vi "Set_Setting.vi"(5 "ChangeonFly":T4, 8 "SettingsCluster":T2={"Sample Rate (us)"=1, "Samples Per Data Point (int, power of 2)"=1000, "DistanceToBulk (um)"=-1.0, "HoldTimeScaler"=1, "SaveData"=TRUE, "DistanceToBulk (um) 2"=-1.0, "DistanceToBulk (um) 3"=-1.0}, 9 "VelScallerCluster":T3, 11 "FPGA VI Reference Out 2":T1) -> (0 "FPGAAccumulatorLength_inpowersof2":i16, 3 "FPGA VI Reference Out 4":T1)   [LabVIEW 2023]
uses:
  TypeDefs/ChangeOnFly.ctl
  TypeDefs/VelScallerCluster.ctl
  TypeDefs/Settings.ctl
  TypeDefs/FPGA VI reference.ctl
  User_Vi/Settings.vi
  <vilib>/Utility/error.llb/Error Cluster From Error Code.vi
  <vilib>/rvi/errors/niLvFpgaAdjustHostInterfaceError.vi
  <vilib>/rvi/interface/nirviReadWriteControl/nirviReadWriteControl.xnode
  FPGA Bitfiles/wecspmpcie7856mi_FPGATarget2_FPGATargetPCIe78_PFpA9M1zUPQ.lvbitx
  NiFpgaLv.dll
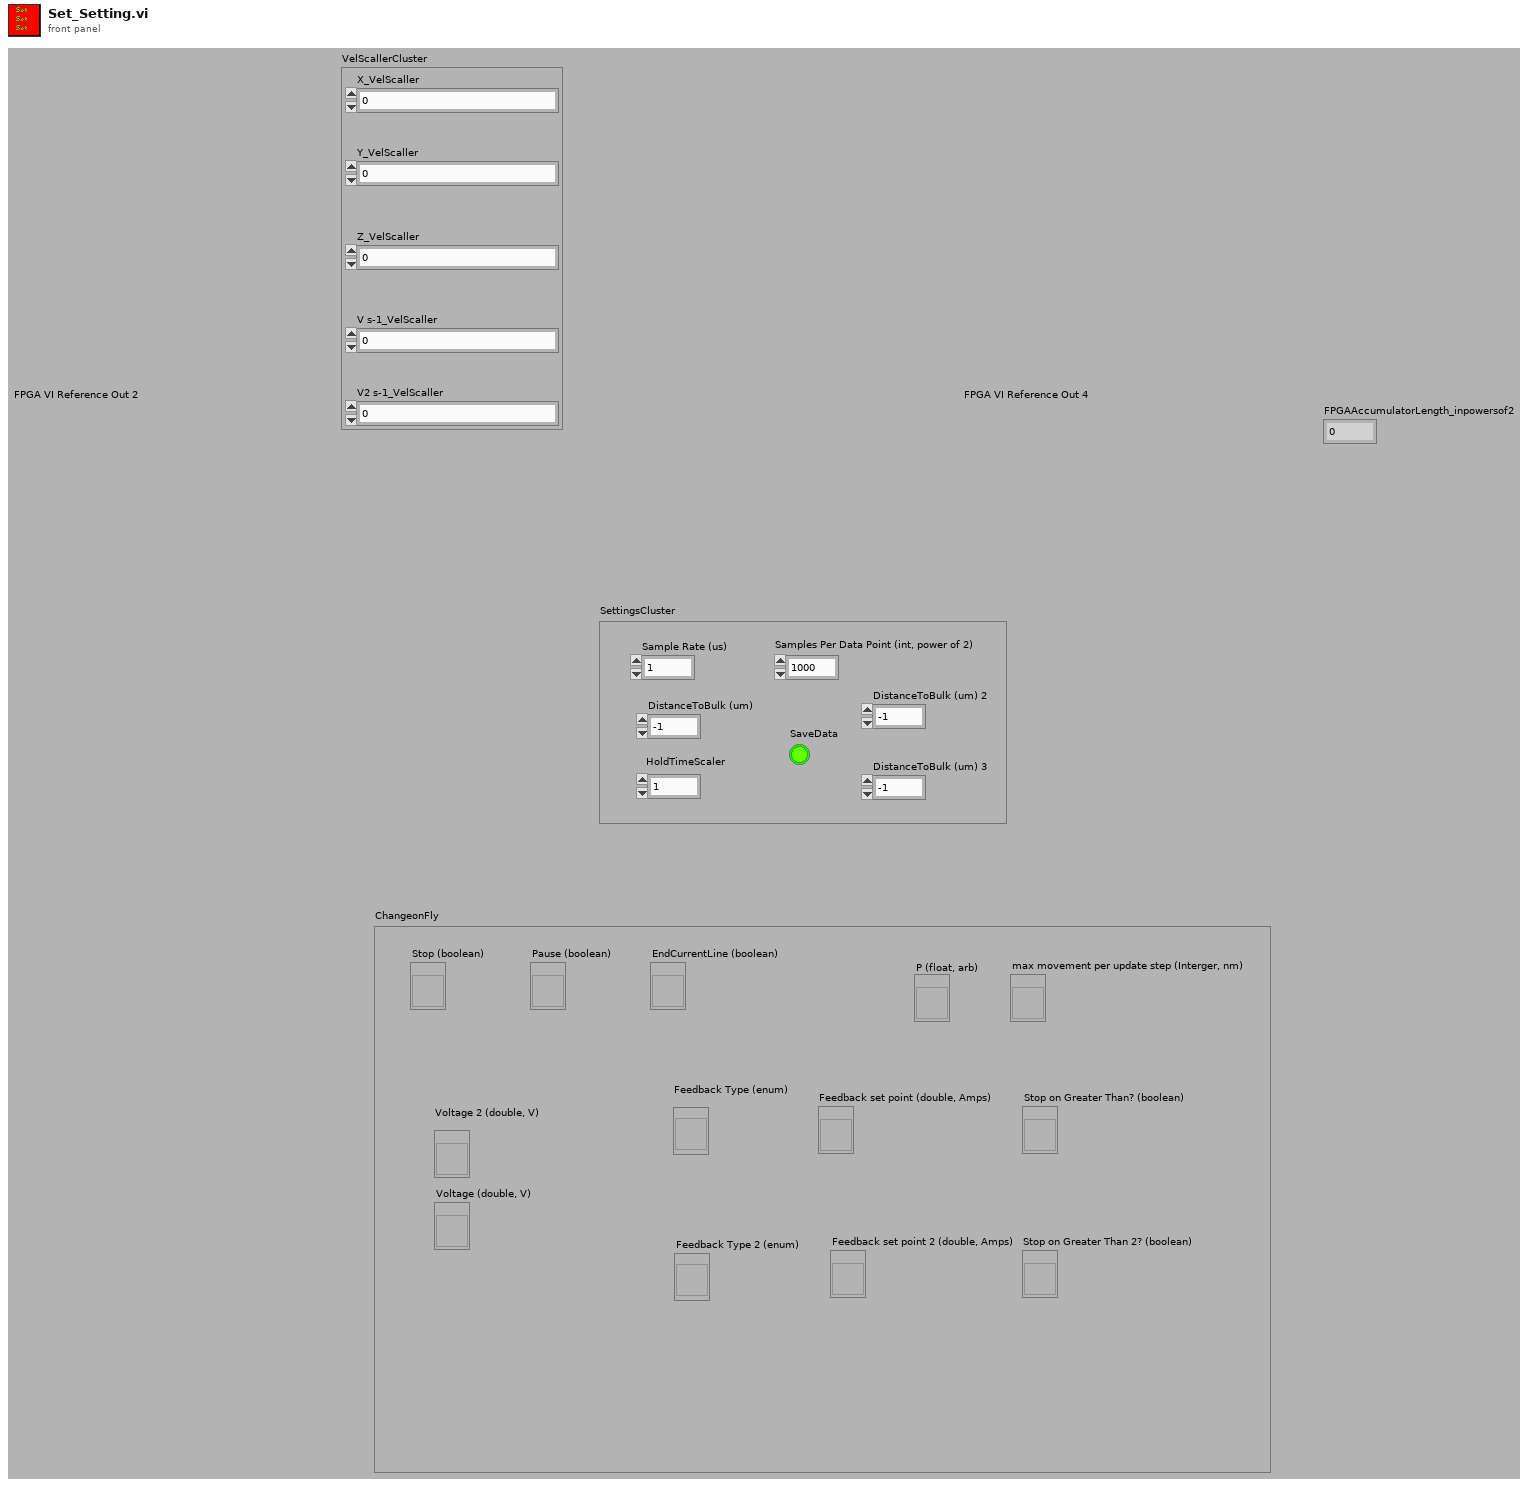
[diagram p1: front panel]
types:
  T1 = typedef "FPGA VI reference.ctl" = refnum<k20>
  T2 = typedef "Settings.ctl" = cluster{"Sample Rate (us)":u32, "Samples Per Data Point (int, power of 2)":i16, "DistanceToBulk (um)":dbl, "HoldTimeScaler":u64, "SaveData":bool, "DistanceToBulk (um) 2":dbl, "DistanceToBulk (um) 3":dbl}
  T3 = typedef "VelScallerCluster.ctl" = cluster{"X_VelScaller":i32, "Y_VelScaller":i32, "Z_VelScaller":i32, "V s-1_VelScaller":i32, "V2 s-1_VelScaller":i32}
  T4 = typedef "ChangeOnFly.ctl" = cluster{"Stop (boolean)":refnum<vi>, "Pause (boolean)":refnum<vi>, "EndCurrentLine (boolean)":refnum<vi>, "max movement per update step (Interger, nm)":refnum<vi>, "P (float, arb)":refnum<vi>, "Feedback set point (double, Amps)":refnum<vi>, "Voltage (double, V)":refnum<vi>, "Feedback set point 2 (double, Amps)":refnum<vi>, "Stop on Greater Than 2? (boolean)":refnum<vi>, "Stop on Greater Than? (boolean)":refnum<vi>, "Voltage 2 (double, V)":refnum<vi>, "Feedback Type (enum)":refnum<vi>, "Feedback Type 2 (enum)":refnum<vi>}
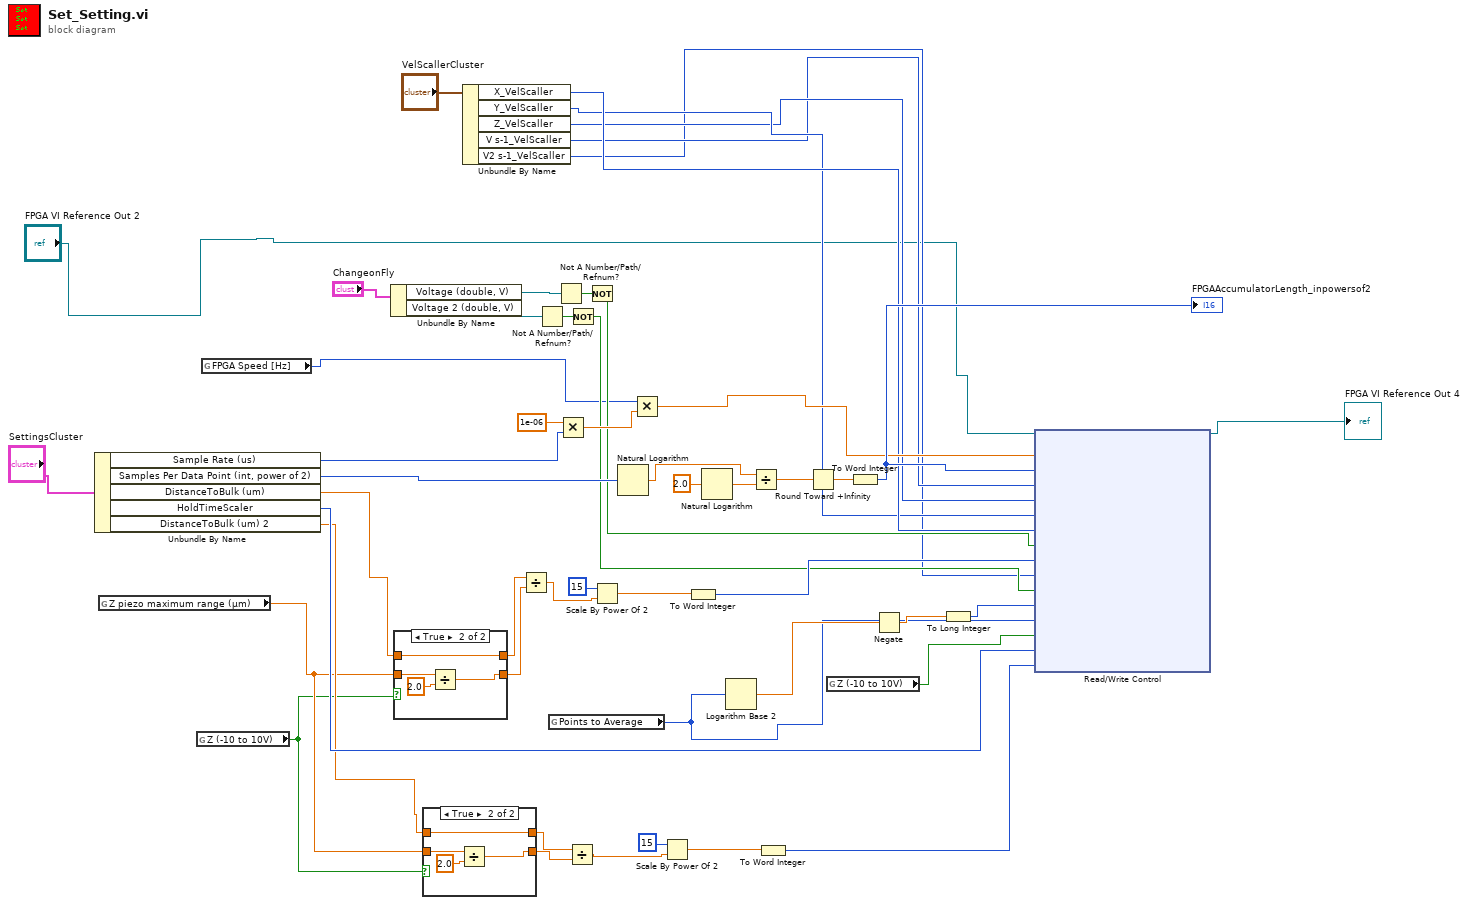
[diagram p0: block diagram]
diagram:
  n1 = Unbundle By Name("SettingsCluster") -> ("Sample Rate (us)"=w40:u32, "Samples Per Data Point (int, power of 2)"=w49:i16, "DistanceToBulk (um)"=w26:dbl, "HoldTimeScaler"=w15:u64, "DistanceToBulk (um) 2"=w9:dbl)
  n2 = global read "Settings.vi" "Z piezo maximum range (µm)"() -> (w8:dbl)
  n3 = global read "Settings.vi" "Z (-10 to 10V)"() -> (w7:bool)
  n4 = global read "Settings.vi" "FPGA Speed [Hz]"() -> (w14:i64)
  n5 = Unbundle By Name("ChangeonFly") -> ("Voltage (double, V)"=w34:refnum<vi>, "Voltage 2 (double, V)"=w30:refnum<vi>)
  n6 = case shown="True" w7 {
    tunnel: w26 -> [w52 w53]
    tunnel: [w52 w53] -> w25
    tunnel: [w51 w54] -> w24
    tunnel: w8 -> [w51 w55]
    frame False {
    }
    frame True {
      n7 = Divide(x=w55, y=2.0) -> (x/y=w54:dbl)
    }
  }
  n8 = case shown="True" w7 {
    tunnel: w9 -> [w58 w59]
    tunnel: [w58 w59] -> w11
    tunnel: [w57 w60] -> w10
    tunnel: w8 -> [w57 w61]
    frame False {
    }
    frame True {
      n9 = Divide(x=w61, y=2.0) -> (x/y=w60:dbl)
    }
  }
  n10 = Unbundle By Name("VelScallerCluster") -> ("X_VelScaller"=w21:i32, "Y_VelScaller"=w20:i32, "Z_VelScaller"=w19:i32, "V s-1_VelScaller"=w18:i32, "V2 s-1_VelScaller"=w17:i32)
  n11 = Divide(x=w25, y=w24) -> (x/y=w41:dbl)
  n12 = Not A Number/Path/Refnum?(number/path/refnum=w30) -> (NaN/Path/Refnum?=w31:bool)
  n13 = global read "Settings.vi" "Points to Average"() -> (w13:u16)
  n14 = Not A Number/Path/Refnum?(number/path/refnum=w34) -> (NaN/Path/Refnum?=w35:bool)
  n15 = Multiply(x=1e-06, y=w40) -> (x*y=w39:dbl)
  n16 = Divide(x=w11, y=w10) -> (x/y=w4:dbl)
  n17 = Not(x=w31) -> (.not. x?=w29:bool)
  n18 = Not(x=w35) -> (.not. x?=w33:bool)
  n19 = Scale By Power Of 2(n=15, x=w41) -> (x*2^n=w43:dbl)
  n20 = Natural Logarithm(1:w49) -> (0:w44:dbl)
  n21 = Multiply(x=w14, y=w39) -> (x*y=w37:dbl)
  n22 = Scale By Power Of 2(n=15, x=w4) -> (x*2^n=w6:dbl)
  n23 = To Word Integer(number=w43) -> (16bit integer=w32:i16)
  n24 = Natural Logarithm(1:2.0 ("x")) -> (0:w45:dbl)
  n25 = Logarithm Base 2(1:w13) -> (0:w28:dbl)
  n26 = Divide(x=w44, y=w45) -> (x/y=w47:dbl)
  n27 = To Word Integer(number=w6) -> (16bit integer=w3:i16)
  n28 = Round Toward +Infinity(x=w47) -> (ceil(x): smallest int >= x=w48:dbl)
  n29 = global read "Settings.vi" "Z (-10 to 10V)"() -> (w12:bool)
  n30 = To Word Integer(number=w48) -> (16bit integer=w50:i16)
  "FPGAAccumulatorLength_inpowersof2" <- w50
  n31 = Negate(x=w28) -> (-x=w23:dbl)
  n32 = To Long Integer(number=w23) -> (32bit integer=w27:i32)
  n33 = xnode ("Read/Write Control")("FPGA VI Reference In"="FPGA VI Reference Out 2", "Buffer Loop Wait Time (tICKS)"=w37, "2^(-n)"=w50, "ExpandVelScaller V"=w18, "ExpandVelScaller Z"=w19, "ExpandVelScaller Y"=w20, "ExpandVelScaller X"=w21, "Change V on Fly"=w33, "DistanceToBulk"=w32, "ExpandVelScaller V2"=w17, "Change V on Fly 2"=w29, "P2AvgMinus"=w27, "P2AvgWhole"=w13, "Z_axis_-10Vto10V"=w12, "HoldTimerScale"=w15, "DistanceToBulk 2"=w3) -> ("FPGA VI Reference Out"=→"FPGA VI Reference Out 4":T1)  [unwired: 1 in, 1 out]
